vi "Onda Trapezoidal.vi"(4 "Informação\nde amostragem":cluster{"Fs":dbl, "#s":dbl}, 6 "Fase (Graus)":dbl, 7 "Reset do sinal":bool, 8 "Entrada de erro":errorcluster, 9 "Amplitude":dbl, 10 "Frequência":dbl, 11 "Offset":dbl) -> (0 "Saída de erro":errorcluster, 3 "Saída de sinal":waveform(dbl))   [LabVIEW 2019]
uses:
  <vilib>/measure/NI_MABase.lvlib
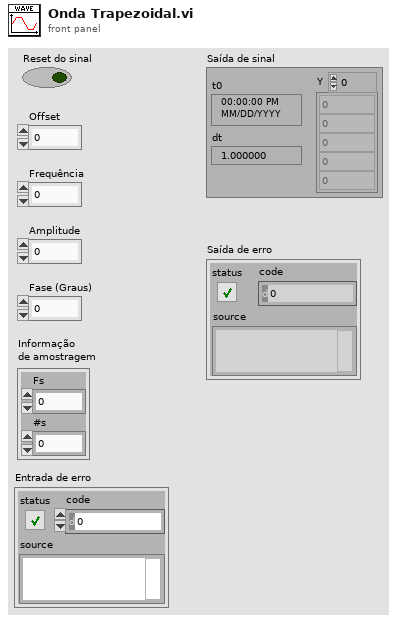
[diagram p1: front panel]
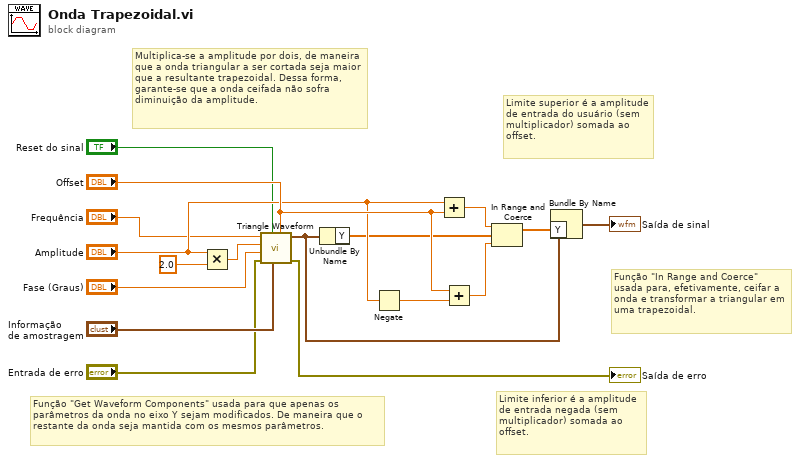
[diagram p0: block diagram]
diagram:
  # "Função \"In Range and Coerce\" usada para, efetivamente, ceifar a onda e transformar a triangular em uma trapezoidal."
  # "Função \"Get Waveform Components\" usada para que apenas os parâmetros da onda no eixo Y sejam modificados. De maneira que o restante da onda seja mantida com os mesmos parâmetros."
  # "Limite inferior é a amplitude de entrada negada (sem multiplicador) somada ao offset."
  # "Limite superior é a amplitude de entrada do usuário (sem multiplicador) somada ao offset."
  # "Multiplica-se a amplitude por dois, de maneira que a onda triangular a ser cortada seja maior que a resultante trapezoidal. Dessa forma, garante-se que a onda ceifada não sofra diminuição da amplitude."
  n1 = Multiply(x="Amplitude", y=2.0) -> (x*y=w11:dbl)
  n2 = call <vilib>:"Triangle Waveform.vi"("offset"="Offset", "sampling info"="Informação\nde amostragem", "reset signal"="Reset do sinal", "error in (no error)"="Entrada de erro", "phase"="Fase (Graus)", "amplitude"=w11, "frequency"="Frequência") -> ("error out"=→"Saída de erro":errorcluster, "signal out"=w9:waveform(dbl))  [unwired: 3 in]
  n3 = Unbundle By Name(w9) -> ("Y"=w7:dbl[])
  n4 = Negate(x="Amplitude") -> (-x=w16:dbl)
  n5 = Add(x="Amplitude", y="Offset") -> (x+y=w13:dbl)
  n6 = Add(x="Offset", y=w16) -> (x+y=w17:dbl)
  n7 = In Range and Coerce(upper limit=w13, x=w7, lower limit=w17) -> (coerced(x)=w8:dbl[])  [unwired: 1 out]
  n8 = Bundle By Name(cluster=w9, "Y"=w8) -> (→"Saída de sinal":waveform(dbl))
